vi "SB get tug location.vi"(2 "Tug":string="L", 3 "Nav String":string="$,G,43,13,230,P,10,20,120,T,10,10,330,L,14,36,110,A,3,5,B,7,8,C,16,20,D,-1,-1,S,08,12,234\r") -> (0 "Valid ?":bool, 1 "Tug Nav Data":cluster{"y":i32, "y":i32})   [LabVIEW 2013]
doc: "This VI gets the location for the Tug specified along with the time data for the data."
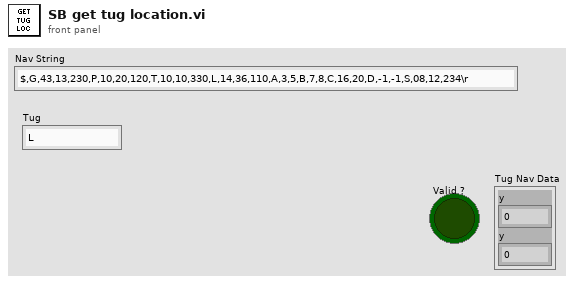
[diagram p1: front panel]
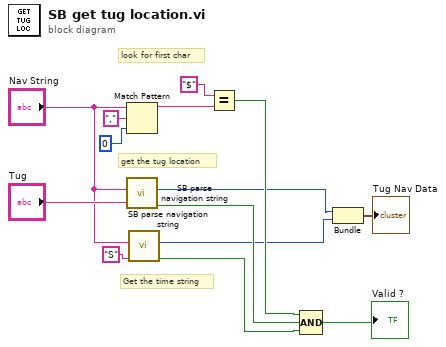
[diagram p0: block diagram]
diagram:
  # "get the tug location"
  # "Get the time string"
  # "look for first char"
  n1 = Match Pattern(string="Nav String", regular expression=",", offset (0)=0) -> (before substring=w13:string)  [unwired: 3 out]
  n2 = call "SB parse navigation string.vi"("Header"="Tug", "Nav String"="Nav String") -> ("Valid?"=w7:bool, "y"=w4:i32)  [unwired: 4 in, 2 out]
  n3 = call "SB parse navigation string.vi"("Header"="S", "Nav String"="Nav String") -> ("Valid?"=w6:bool, "y"=w3:i32)  [unwired: 4 in, 2 out]
  n4 = Equal?(x="$", y=w13) -> (x = y?=w8:bool)
  n5 = Compound Arithmetic op=AND(w8, w7, w6) -> (→"Valid ?":bool)
  n6 = Bundle("y"=w4, "y"=w3) -> (→"Tug Nav Data":cluster{"y":i32, "y":i32})  [unwired: 1 in]
